vi "oa_Check Segment.vi"(0 "X axis selection":u16(ring)=2 items=["Time", "Revolution", "RPM"], 1 "reset?(F)":bool, 7 "segment position":cluster{"start":dbl, "end":dbl, "step size":dbl} {"step size" format="%.2f"; "end" min=0.0 format="%.2f"; "start" min=0.0 format="%.2f"}, 9 "speed profile":T1 {"speed [RPM]" format="%.2f"; "time [s]" format="%.2f"}, 11 "error in (no error)":errorcluster) -> (3 "reset out":bool, 4 "X axis selection":u16(ring)=2 items=["Time", "Revolution", "RPM"], 6 "step found?":bool, 8 "segment position out":cluster{"start":dbl, "end":dbl, "step size":dbl} {"step size" format="%.2f"; "end" min=0.0 format="%.2f"; "start" min=0.0 format="%.2f"}, 10 "dul speed profile":T1 {"speed [RPM]" format="%.2f"; "time [s]" format="%.2f"}, 15 "error out":errorcluster)   [LabVIEW 2017]
uses:
  <vilib>/addons/Sound and Vibration/Order Analysis/Tach Process/SubVIs/speed profile.ctl
  <vilib>/addons/Sound and Vibration/Order Analysis/Tach Process/SoundVib_TachProcess.lvlib
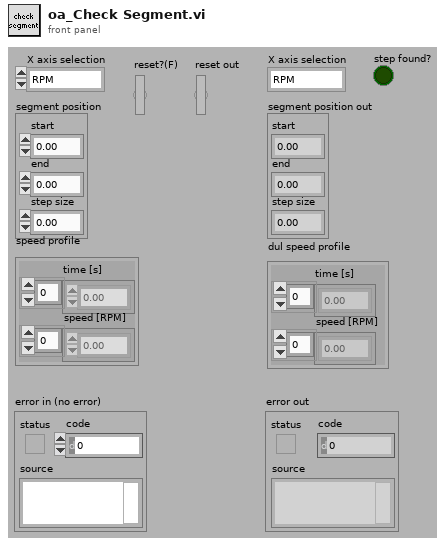
[diagram p1: front panel]
types:
  T1 = typedef "SoundVib_TachProcess.lvlib/speed profile.ctl" = cluster{"time [s]":dbl[], "speed [RPM]":dbl[]}
  T2 = cluster{"start output":dbl, "end output":dbl, "step output":dbl}
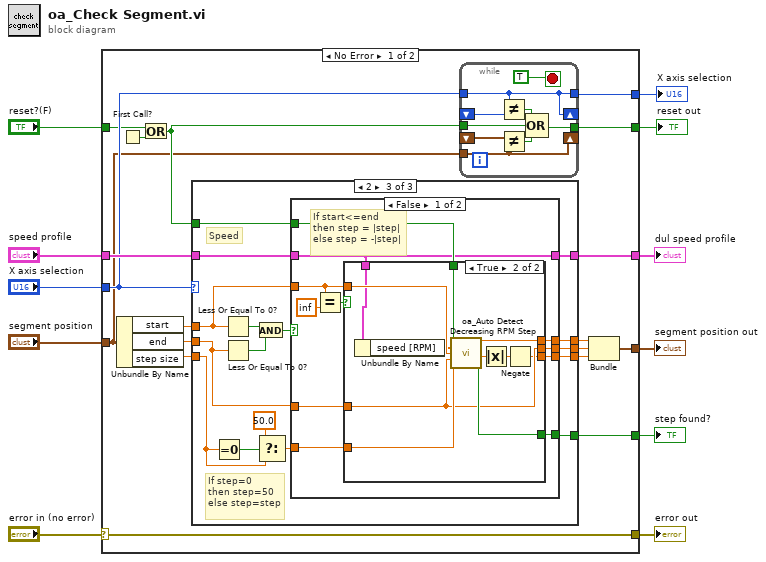
[diagram p0: block diagram]
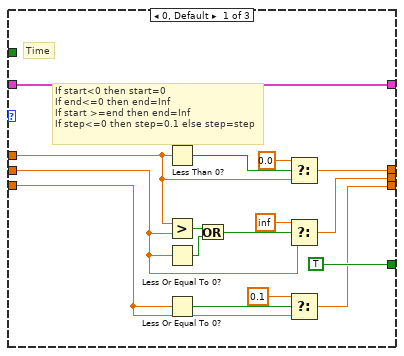
[diagram p2: hidden frame]
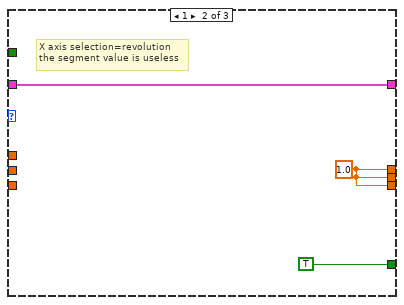
[diagram p3: hidden frame]
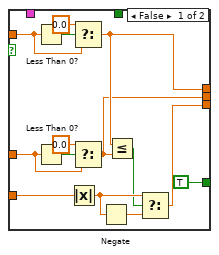
[diagram p4: hidden frame]
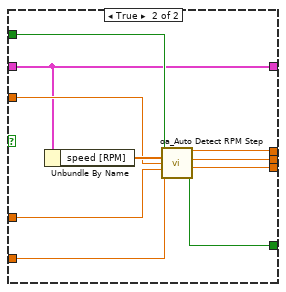
[diagram p5: hidden frame]
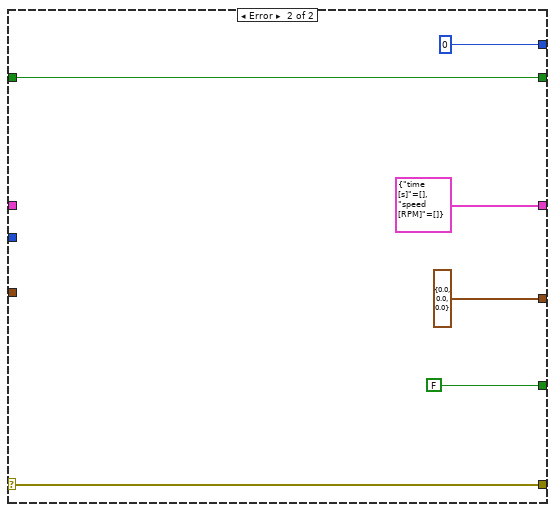
[diagram p6: hidden frame]
diagram:
  n1 = case shown="No Error" "error in (no error)" {
    selector: "error in (no error)" -> [w29 w125]
    tunnel: [w29 w125] -> w10
    tunnel: "X axis selection" -> [w21 _]
    tunnel: "segment position" -> [w12 _]
    tunnel: [w13 cluster{"start":dbl, "f":dbl, "step size":dbl} {"start"=0.0, "f"=0.0, "step size"=0.0}] -> w7
    tunnel: [w25 FALSE ("step found?")] -> w6
    tunnel: [w24 T1 {"time [s]"=[], "speed [RPM]"=[]} ("speed profile")] -> w4
    tunnel: "speed profile" -> [w23 _]
    tunnel: "reset?(F)" -> [w20 w120]
    tunnel: [w18 u16 0 ("segment unit")] -> w2
    tunnel: [w16 w120] -> w1
    frame No Error {
      n2 = Unbundle By Name(w12) -> ("start"=w28:dbl, "end"=w27:dbl, "step size"=w26:dbl)
      n3 = First Call?() -> (First Call?: T/F=w17:bool)
      n4 = Or(x=w20, y=w17) -> (x .or. y?=w19:bool)
      n5 = case shown="2" w21 {
        tunnel: w28 -> [w49 _ w61]
        tunnel: w27 -> [w45 _ w62]
        tunnel: w26 -> [w46 _ w63]
        tunnel: [TRUE ("step found?") TRUE ("step found?") w65] -> w25
        tunnel: [w43 w57 w67] -> w24
        tunnel: w23 -> [w43 w57 w66]
        tunnel: [w42 w55 w70] -> w22
        tunnel: [w41 w55 w69] -> w15
        tunnel: [w40 w55 w68] -> w14
        tunnel: w19 -> [_ _ w64]
        frame 0, Default {
          # "Time"
          # "If start<0 then start=0\nIf end<=0 then end=Inf\nIf start >=end then end=Inf\nIf step<=0 then step=0.1 else step=step"
          n6 = Less Than 0?(x=w49) -> (x < 0?=w39:bool)
          n7 = Greater?(x=w49, y=w45) -> (0:w54:bool)
          n8 = Less Or Equal To 0?(x=w45) -> (x <= 0?=w52:bool)
          n9 = Less Or Equal To 0?(x=w46) -> (x <= 0?=w48:bool)
          n10 = Or(x=w54, y=w52) -> (x .or. y?=w53:bool)
          n11 = Select(t=0.0, s=w39, f=w49) -> (s? t:f=w42:dbl)
          n12 = Select(t=inf ("f"), s=w53, f=w45) -> (s? t:f=w41:dbl)
          n13 = Select(t=0.1, s=w48, f=w46) -> (s? t:f=w40:dbl)
        }
        frame 1 {
          w55 = 1.0 ("start output")
          # "X axis selection=revolution\nthe segment value is useless"
        }
        frame 2 {
          # "If step=0\nthen step=50\nelse step=step"
          # "Speed"
          n14 = Equal To 0?(x=w63) -> (x = 0?=w73:bool)
          n15 = Less Or Equal To 0?(x=w61) -> (x <= 0?=w60:bool)
          n16 = Less Or Equal To 0?(x=w62) -> (x <= 0?=w59:bool)
          n17 = And(x=w60, y=w59) -> (x .and. y?=w58:bool)
          n18 = Select(t=50.0, s=w73, f=w63) -> (s? t:f=w71:dbl)
          n19 = case shown="False" w58 {
            tunnel: w61 -> [w78 w117]
            tunnel: w62 -> [w81 w116]
            tunnel: w71 -> [w84 w115]
            tunnel: [w80 w114] -> w70
            tunnel: [w79 w113] -> w69
            tunnel: [w83 w112] -> w68
            tunnel: [w74 w110] -> w67
            tunnel: w66 -> [w74 w110]
            tunnel: [w82 w111] -> w65
            tunnel: w64 -> [w75 w119]
            frame False {
              # "If start<=end\nthen step = |step|\nelse step = -|step|"
              n20 = Equal?(x=w78, y=inf) -> (x = y?=w76:bool)
              n21 = case shown="True" w76 {
                tunnel: w84 -> [w98 w106]
                tunnel: [w95 w99] -> w83
                tunnel: [TRUE ("step found?") w107] -> w82
                tunnel: w78 -> [w91 w105]
                tunnel: w81 -> [w88 w101]
                tunnel: [w86 w109] -> w80
                tunnel: [w85 w101] -> w79
                tunnel: w75 -> [_ w104]
                tunnel: w74 -> [_ w103]
                frame False {
                  n22 = Less Than 0?(x=w91) -> (x < 0?=w93:bool)
                  n23 = Less Than 0?(x=w88) -> (x < 0?=w89:bool)
                  n24 = Absolute Value(x=w98) -> (abs(x)=w97:dbl)
                  n25 = Select(t=0.0, s=w93, f=w91) -> (s? t:f=w86:dbl)
                  n26 = Select(t=0.0, s=w89, f=w88) -> (s? t:f=w85:dbl)
                  n27 = Negate(x=w97) -> (-x=w96:dbl)
                  n28 = Less Or Equal?(x=w86, y=w85) -> (x <= y?=w87:bool)
                  n29 = Select(t=w97, s=w87, f=w96) -> (s? t:f=w95:dbl)
                }
                frame True {
                  n30 = Unbundle By Name(w103) -> ("speed [RPM]"=w102:dbl[])
                  n31 = call <vilib>:"oa_Auto Detect Decreasing RPM Step.vi"("reset?"=w104, "speed(RPM)"=w102, "start input"=w105, "end input"=w101, "step input"=w106) -> ("start output"=w109:dbl, "step output"=w108:dbl, "step found?"=w107:bool)  [unwired: 7 in, 1 out]
                  n32 = Absolute Value(x=w108) -> (abs(x)=w100:dbl)
                  n33 = Negate(x=w100) -> (-x=w99:dbl)
                }
              }
            }
            frame True {
              n34 = Unbundle By Name(w110) -> ("speed [RPM]"=w118:dbl[])
              n35 = call <vilib>:"oa_Auto Detect RPM Step.vi"("reset?"=w119, "speed(RPM)"=w118, "start input"=w117, "end input"=w116, "step input"=w115) -> ("start output"=w114:dbl, "end output"=w113:dbl, "step output"=w112:dbl, "step found?"=w111:bool)  [unwired: 7 in]
            }
          }
        }
      }
      n36 = while {
        shift-right: [w34] -> _
        shift-left: _ -> [w38]
        tunnel: w21 -> [w34]
        tunnel: w19 -> [w35]
        tunnel: [w34] -> w18
        tunnel: [w33] -> w16
        shift-right: [w30] -> _
        shift-left: _ -> [w32]
        tunnel: w12 -> [w30]
        stop <- TRUE stop-if-true
        n37 = Not Equal?(x=w34, y=w38) -> (x != y?=w36:bool)
        n38 = Not Equal?(x=w32, y=w30) -> (x != y?=w31:bool)
        n39 = Compound Arithmetic op=OR(w36, w35, w31) -> (w33:bool)
      }
      n40 = Bundle("start output"=w22, "end output"=w15, "step output"=w14) -> (w13:T2)  [unwired: 1 in]
    }
    frame Error {
    }
  }
  "error out" <- w10
  "segment position out" <- w7
  "step found?" <- w6
  "dul speed profile" <- w4
  "X axis selection" <- w2
  "reset out" <- w1
